vi "pid-toolkit-autotuning.vi"() -> ()   [LabVIEW 2018, in "pid-toolkit.lvlib"]
uses:
  <vilib>/Platform/TimedLoop/XDataNode/timing_clust.ctl
  <vilib>/Platform/TimedLoop/XDataNode/nitl_modes.ctl
  <vilib>/Platform/TimedLoop/XDataNode/wakeup.ctl
  <vilib>/platform/TimedLoop/XDataNode/XDataNode.xnode
  pid-toolkit.lvlib
  <vilib>/Platform/TimedLoop/XDataNode/XDNodeRunTimeDep.lvlib
  <vilib>/addons/control/pid/NI_PID_autopid.lvlib
panel:
  out "tuning completed?":bool
  out "PID gains out":T1={"proportional gain (Kc)"=1.0, "integral time (Ti, min)"=0.01, "derivative time (Td, min)"=0.0} {"derivative time (Td, min)" format="%.3f"; "integral time (Ti, min)" format="%.3f"; "proportional gain (Kc)" format="%.3f"}
  out "output":dbl format="%.2f"
  out "dt out (s)":dbl format="%.3f"
  in  "reinitialize? (F)":bool
  in  "PID gains":T1={"proportional gain (Kc)"=1.0, "integral time (Ti, min)"=0.01, "derivative time (Td, min)"=0.0} {"derivative time (Td, min)" format="%.3f"; "integral time (Ti, min)" format="%.3f"; "proportional gain (Kc)" format="%.3f"}
  out "output range":cluster{"output high":dbl, "output low":dbl}={"output high"=100.0, "output low"=-100.0} {"output low" format="%.2f"; "output high" format="%.2f"}
  in  "autotuning parameters":T2={"controller type"=1, "relay cycles"=3, "relay amplitude"=1.0, "control specification"=2, "PV noise level"=0.1} {"PV noise level" format="%.2f"; "control specification" items=["normal", "fast", "slow"]; "relay amplitude" format="%.2f"; "controller type" items=["PID", "PI", "P"]}
  out "Plot":T3(graph)
  in  "autotune? (F)":bool
  out "Output":u16
  out "High":bool
  out "Low":bool
  in  "Setpoint":dbl(slide) scale=0.0..100.0
  out "Modbus error":errorcluster
  in  "Off Hook":bool
  in  "Update Rate":dbl caption="Rate"
  out "Failure":bool
  out "Updating":bool
  in  "Update Now":bool
  in  "Maximum":sgl
  in  "Minimum":sgl
  out "Thermometer":sgl(slide) scale=0.0..260.0
  in  "Force exit out of loop":bool
  out "Interval":i64
  out "Duration":i64
  out "Cycle":i32
  in  "Frequency":dbl(slide) scale=0.1..10.0
  # "Loop"
  # "Modbus"
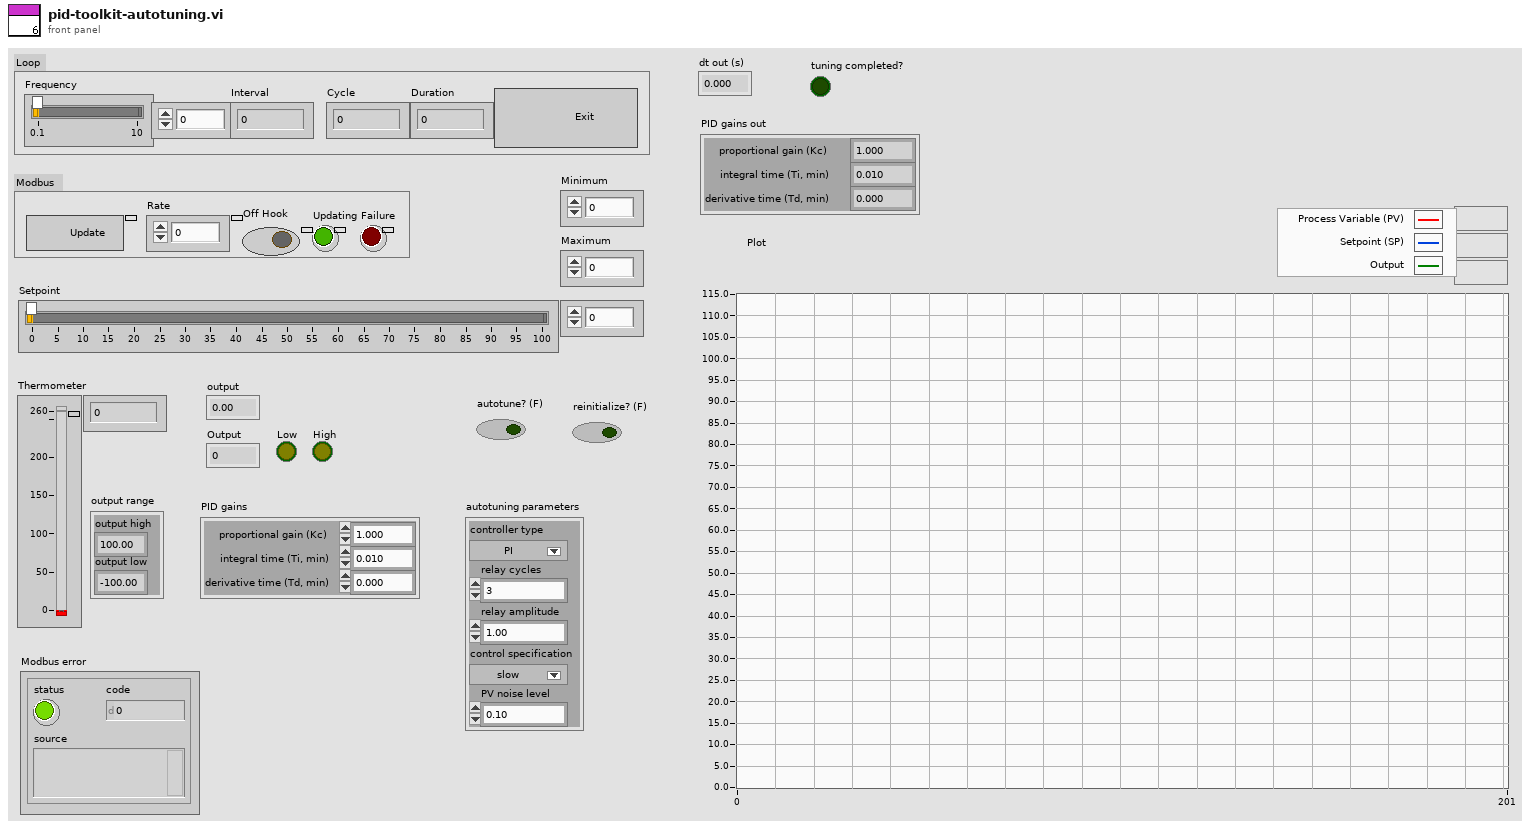
[diagram p1: front panel]
types:
  T1 = cluster{"proportional gain (Kc)":dbl, "integral time (Ti, min)":dbl, "derivative time (Td, min)":dbl}
  T2 = cluster{"controller type":u16, "relay cycles":i32, "relay amplitude":dbl, "control specification":u16, "PV noise level":dbl}
  T3 = cluster{dbl, "desired temperature":dbl, "output":dbl}
  T4 = typedef "XDNodeRunTimeDep.lvlib/timing_clust.ctl" = cluster{"Expected End [f-1]":u64, "Actual End [f-1]":u64, "Finished Late? [f-1]":bool, "Expected End [i-1]":u64, "Actual End [i-1]":u64, "Finished Late? [i-1]":bool, "Expected Start [i]":u64, "Actual Start [i]":u64, "Expected Start [f]":u64, "Actual Start [f]":u64, "Source Name":string, "Structure Name":string, "Period":i64, "Deadline":i64, "Offset":i64, "Start":i64, "Priority":i32, "Timeout":i32, "Mode":T5, "Wakeup Reason":T6, "Error":errorcluster, "Source Type":string, "Secondary Source Type":string, "Global End Time":u64, "Global Start Time":u64, "Frame Duration":u64, "Iteration Duration":u64, "Assigned CPU":i32, "I/O Scan Engine Mode":u32}
  T5 = typedef "XDNodeRunTimeDep.lvlib/nitl_modes.ctl" = enum32{"No Change", "Process missed periods, maintain original phase", "Discard missed periods, maintain original phase", "Process missed periods, ignore original phase", "Discard missed periods, ignore original phase"}
  T6 = typedef "XDNodeRunTimeDep.lvlib/wakeup.ctl" = enum32{"Normal", "Aborted", "Asynchronous wakeup", "Timing source error", "Timed loop error", "Timeout"}
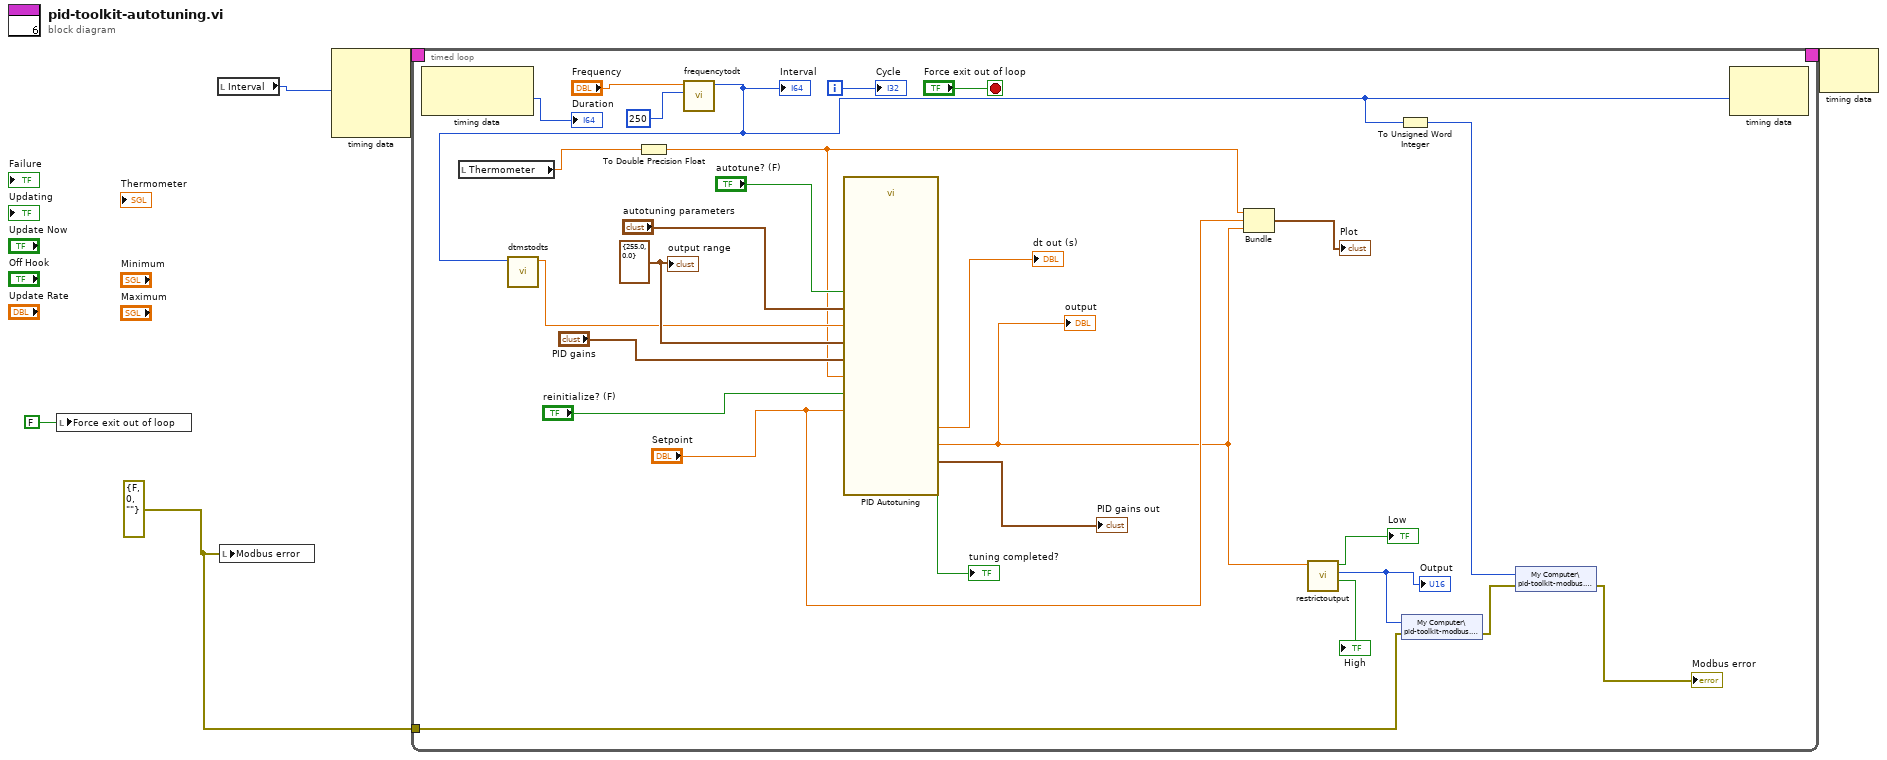
[diagram p0: block diagram]
diagram:
  w1 = errorcluster {"status"=FALSE, "code"=0, "source"=""} ("Modbus error")
  n1 = local write "Force exit out of loop"(FALSE ("Force exit out of loop")) -> ()
  n2 = local read "Interval"() -> (w2:i64)
  n3 = local write "Modbus error"(w1) -> ()
  n4 = node-c288(w2) -> (w5:T4)  [unwired: 3 in]
  n5 = timed-loop {
    timing: w5 -> [_]
    timing-out: [_] -> w4
    tunnel: w1 -> [w27]
    i -> [w28]
    stop <- "Force exit out of loop" stop-if-true
    w9 = cluster{"output high":dbl, "output low":dbl} {"output high"=255.0, "output low"=0.0} ("output range")
    n6 = node-c288() -> (→"Duration":i64)  [unwired: 1 in, 1 out]
    n7 = local read "Thermometer"() -> (w18:sgl)
    n8 = To Double Precision Float(number=w18) -> (double precision float=w7:dbl)
    n9 = call "frequencytodt.vi"("Default in"=i64 250, "Frequency"="Frequency") -> ("Default out"=w20:i64)  [unwired: 9 in]
    "Interval" <- w20
    n10 = call "dtmstodts.vi"("Default in"=w20) -> ("Numeric"=w8:dbl)  [unwired: 10 in]
    n11 = call <vilib>:"PID Autotuning.vi"("autotune? (F)"="autotune? (F)", "autotuning parameters"="autotuning parameters", "reinitialize? (F)"="reinitialize? (F)", "output range"=w9, "dt (s)"=w8, "PID gains"="PID gains", "process variable"=w7, "setpoint"="Setpoint") -> ("dt out (s)"=→"dt out (s)":dbl, "PID gains out"=→"PID gains out":T1, "tuning completed?"=→"tuning completed?":bool, "output"=w11:dbl)
    "output" <- w11
    n12 = Bundle(w7, "Setpoint"="Setpoint", "output"=w11) -> (→"Plot":cluster{dbl, "Setpoint":dbl, "output":dbl})  [unwired: 1 in]
    n13 = call "restrictoutput.vi"("Input"=w11) -> ("Hig"=→"High":bool, "Output"=w24:u16, "Low"=→"Low":bool)  [unwired: 8 in]
    "Output" <- w24
    n14 = To Unsigned Word Integer(number=w20) -> (unsigned 16bit integer=w21:u16)
    n15 = shared-variable "My Computer\\pid-toolkit-modbus.lvlib\\400002"(w24, error in=w27) -> (error out=w23:errorcluster)
    n16 = shared-variable "My Computer\\pid-toolkit-modbus.lvlib\\400001"(w21, error in=w23) -> (error out=→"Modbus error":errorcluster)
    n17 = node-c288(w20) -> ()  [unwired: 1 in, 1 out]
    "Cycle" <- w28
    "output range" <- w9
  }
  n18 = node-c288(w4) -> ()  [unwired: 1 out]
